vi "Split String.vi"(8 "error in (no error)":errorcluster, 9 "Post Split":string, 10 "Pre Split":string, 11 "Path in":path) -> (0 "error out":errorcluster, 2 "Formatted name":string, 3 "Dup Path out":path)   [LabVIEW 2019, in "AutoMenuCreator.lvlib"]
uses:
  AutoMenuCreator.lvlib
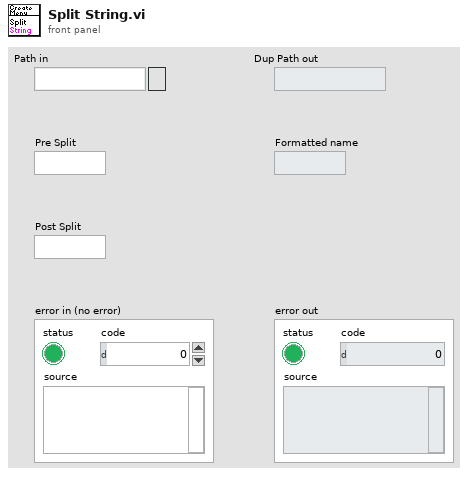
[diagram p1: front panel]
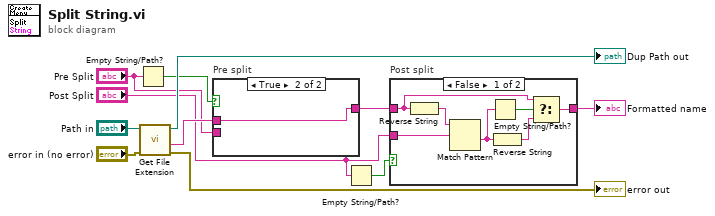
[diagram p0: block diagram]
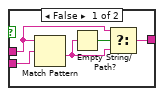
[diagram p3: hidden frame]
diagram:
  n1 = Empty String/Path?(string/path="Pre Split") -> (empty?=w6:bool)
  n2 = call <vilib>:"Get File Extension.vi"("error in (no error)"="error in (no error)", "file"="Path in") -> ("error out"=→"error out":errorcluster, "filename without extension"=w9:string, "dup file"=→"Dup Path out":path)  [unwired: 5 in, 2 out]
  n3 = case "Pre split" shown="True" w6 {
    tunnel: [w16 w17] -> w3
    tunnel: w9 -> [w14 w17]
    tunnel: "Pre Split" -> [w12 _]
    frame False {
      n4 = Match Pattern(string=w14, regular expression=w12) -> (after substring=w15:string)  [unwired: 1 in, 3 out]
      n5 = Empty String/Path?(string/path=w15) -> (empty?=w13:bool)
      n6 = Select(t=w14, s=w13, f=w15) -> (s? t:f=w16:string)
    }
    frame True {
    }
  }
  n7 = Empty String/Path?(string/path="Post Split") -> (empty?=w4:bool)
  n8 = case "Post split" shown="False" w4 {
    tunnel: [w18 w25] -> w1
    tunnel: w3 -> [w20 w25]
    tunnel: "Post Split" -> [w22 _]
    frame False {
      n9 = Reverse String(1:w20) -> (0:w21:string)
      n10 = Match Pattern(string=w21, regular expression=w22) -> (after substring=w24:string)  [unwired: 1 in, 3 out]
      n11 = Empty String/Path?(string/path=w24) -> (empty?=w23:bool)
      n12 = Reverse String(1:w24) -> (0:w19:string)
      n13 = Select(t=w20, s=w23, f=w19) -> (s? t:f=w18:string)
    }
    frame True {
    }
  }
  "Formatted name" <- w1
